vi "DigitalRead.vi"(3 "error in (no error)":errorcluster, 4 "Terminal in":u8, 5 "VISA Refnum in":refnum<visa-resource-name>) -> (0 "error out":errorcluster, 1 "element":u8, 2 "VISA Refnum out":refnum<visa-resource-name>)   [LabVIEW 2016]
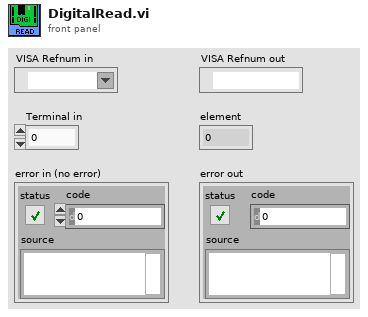
[diagram p1: front panel]
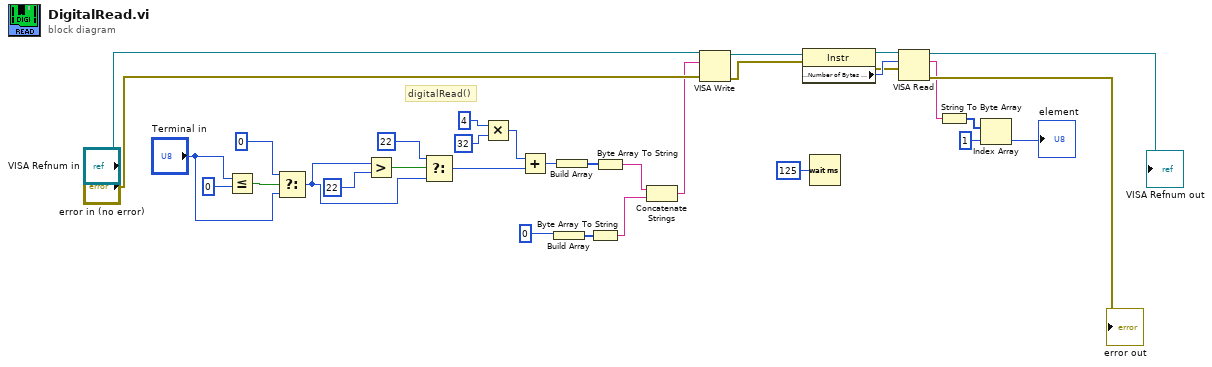
[diagram p0: block diagram]
diagram:
  # "digitalRead()"
  n1 = Less Or Equal?(x="Terminal in", y=u8 0) -> (x <= y?=w12:bool)
  n2 = Select(t=u8 0, s=w12, f="Terminal in") -> (s? t:f=w9:u8)
  n3 = Greater?(x=w9, y=u8 22) -> (0:w17:bool)
  n4 = Select(t=u8 22, s=w17, f=w9) -> (s? t:f=w1:u8)
  n5 = Multiply(x=u8 4, y=u8 32) -> (x*y=w14:u8)
  n6 = Add(x=w14, y=w1) -> (x+y=w8:u8)
  n7 = Build Array(u8 0) -> (w6:u8[])
  n8 = Build Array(w8) -> (w7:u8[])
  n9 = Byte Array To String(unsigned byte array=w6) -> (string=w5:string)
  n10 = Byte Array To String(unsigned byte array=w7) -> (string=w4:string)
  n11 = Concatenate Strings(w4, w5) -> (w3:string)
  n12 = VISA Write(VISA resource name="VISA Refnum in", write buffer=w3, error in (no error)="error in (no error)") -> (VISA resource name out=w23:refnum<visa-resource-name>, error out=w24:errorcluster)  [unwired: 1 out]
  n13 = property class="Instr"(reference=w23, error in=w24) -> (reference out=w20:refnum<visa-resource-name>, error out=w21:errorcluster, "Serial Settings:Number of Bytes at Serial Port"=w22:u32)
  n14 = Wait (ms)(milliseconds to wait=u32 125) -> ()  [unwired: 1 out]
  n15 = VISA Read(VISA resource name=w20, byte count=w22, error in (no error)=w21) -> (VISA resource name out=→"VISA Refnum out":refnum<visa-resource-name>, read buffer=w2:string, error out=→"error out":errorcluster)  [unwired: 1 out]
  n16 = String To Byte Array(string=w2) -> (unsigned byte array=w30:u8[])
  n17 = Index Array(array=w30, index=1) -> (element=→"element":u8)
